vi "steam.vi"(8 "error in (no error)":errorcluster, 11 "Chef in":refnum<class "Chef.lvclass">) -> (0 "error out":errorcluster, 3 "Chef out":refnum<class "Chef.lvclass">)   [LabVIEW 2020, in "Chef.lvclass"]
uses:
  Chef.lvclass
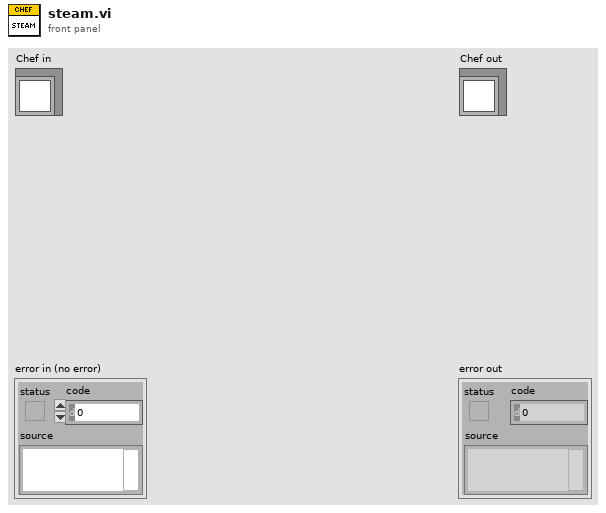
[diagram p1: front panel]
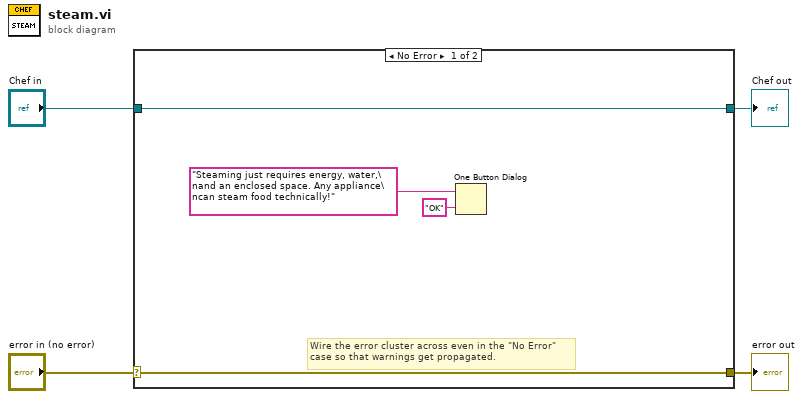
[diagram p0: block diagram]
diagram:
  n1 = case shown="No Error" "error in (no error)" {
    selector: "error in (no error)" -> [w7 w10]
    tunnel: [w7 w10] -> w3
    tunnel: [w8 w9] -> w1
    tunnel: "Chef in" -> [w8 w9]
    frame No Error {
      # "Wire the error cluster across even in the \"No Error\"\ncase so that warnings get propagated."
      n2 = One Button Dialog(message="Steaming just requires energy, water,\nand an enclosed space. Any appliance\ncan steam food technically!", button name ("OK")="OK") -> ()  [unwired: 1 out]
    }
    frame Error {
    }
  }
  "error out" <- w3
  "Chef out" <- w1
